vi "Main.vi"(11 "Module Admin":refnum<class "Delacor_lib_QMH_Module Admin.lvclass">) -> ()   [LabVIEW 2020, in "UI.lvlib"]
doc: "This template is based off of the Queued Message Handler design pattern and the Queued Message Handler project template that ships with LabVIEW.\n\nThe main difference is that the queue is private to this module and communication between modules is performed via Broadcast and Request events.\n\nRequest events are wrapped in public API methods and are handled in the Event Handling Loop (EHL) of this VI. Any module can register for Broadcast events sent by this module. The EHL generates messages based on user interface actions.\n\nThe Message Handling Loop (MHL) processes messages generated by the EHL, or by other messages. The messages are string values, so new messages can be added easily to the Message Cases case structure in the MHL. Each message cluster can also provide an optional value for Message Data, which is a variant that can be converted to whatever message-specific data is required.\n_____\nBased on DQMH Dev Tools: Project Template 7.1.2.1547."
uses:
  UI.lvlib
  <vilib>/Delacor/Delacor QMH/Libraries/Module Admin_class/Delacor_lib_QMH_Module Admin.lvclass
  <vilib>/Delacor/Delacor QMH/Libraries/Message Queue_class/Delacor_lib_QMH_Message Queue.lvclass/Delacor_lib_QMH_Message Queue.ctl
  <vilib>/Delacor/Delacor QMH/Libraries/Module Admin_class/Delacor_lib_QMH_Module Admin.lvclass/Delacor_lib_QMH_Module Admin.ctl
  <vilib>/Delacor/Delacor QMH/Libraries/Message Queue_class/Delacor_lib_QMH_Message Queue.lvclass
  Module Data--cluster.ctl
  <vilib>/Utility/miscctls.llb/LVPointTypeDef.ctl
  <vilib>/Delacor/Delacor QMH/Libraries/Message Queue_class/Delacor_lib_QMH_Enqueue Message (Single).vi
  Stop Argument--cluster.ctl
  Get Analog Data Argument--cluster.ctl
panel:
  out "Value":dbl[](array[numeric])
  in  "Start/Stop":bool
  in  "Close":bool
  in  "DAQmx Analog Channels":tag[](array[tag])
  out "error out":errorcluster
  out "Status":string
  in  "Simulate MHL Error":bool
  in  "Simulate EHL Error":bool
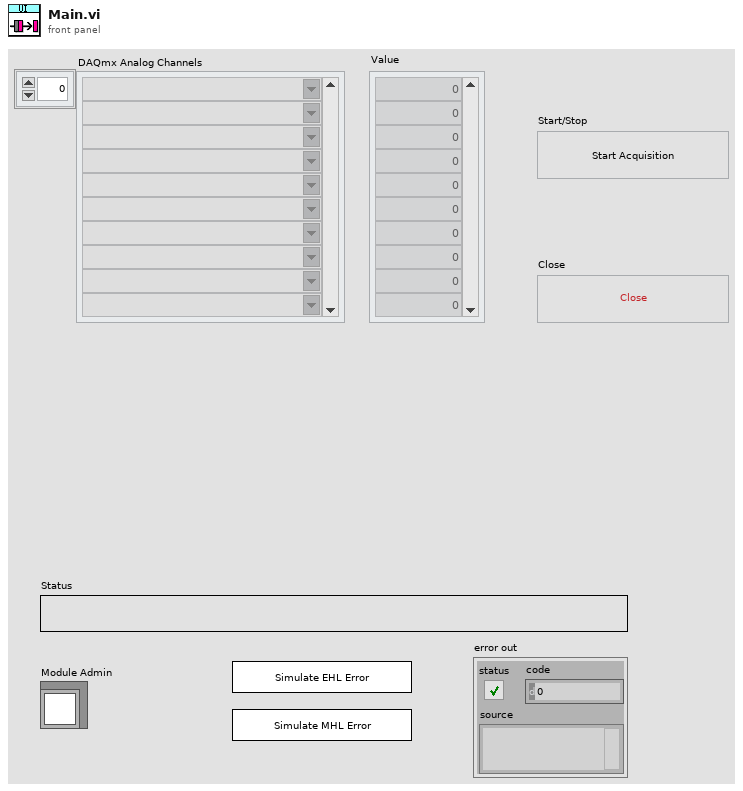
[diagram p1: front panel]
types:
  T1 = typedef "UI.lvlib/Request Events--cluster.ctl" = cluster{"Stop Module":refnum<user-event>, "Show Panel":refnum<user-event>, "Hide Panel":refnum<user-event>, "Get Module Execution Status":refnum<user-event>, "Show Diagram":refnum<user-event>, "Get Analog Data":refnum<user-event>}
  T2 = typedef "UI.lvlib/Module Data--cluster.ctl" = cluster{"Status":string, "Value":dbl[]}
  T3 = enum32{"invalid lock state", "Not Locked", "Locked (No Password)", "Password-protected"}
  T4 = typedef "UI.lvlib/Stop Argument--cluster.ctl" = cluster{"Origin":string, "Exit via Stop Module Req?":bool, "Wait for Module to stop?":bool}
  T5 = typedef "UI.lvlib/Get Analog Data Argument--cluster.ctl" = cluster{"Index":i32, "Value":dbl}
  T6 = enum8{"Enabled", "Disabled", "Disabled and Grayed Out"}
  T7 = typedef "LVPointTypeDef.ctl" = cluster{"Horizontal":i16, "Vertical":i16}
  T8 = enum32{"Invalid", "Standard", "Closed", "Hidden", "Minimized", "Maximized"}
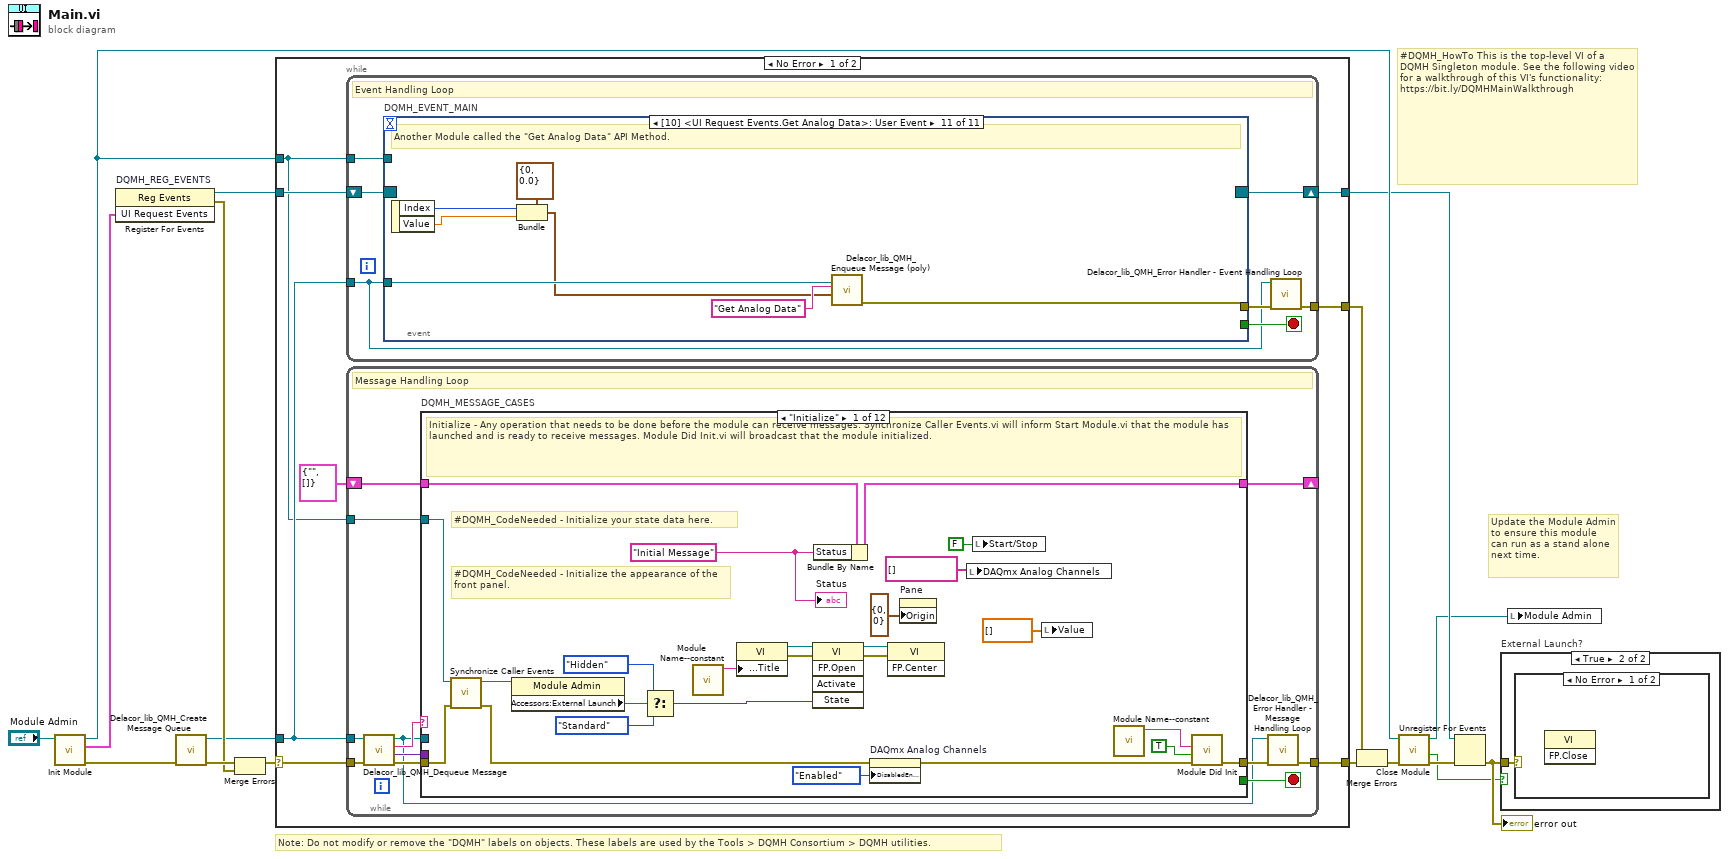
[diagram p0: block diagram]
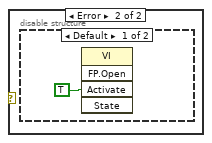
[diagram p3: hidden frame]
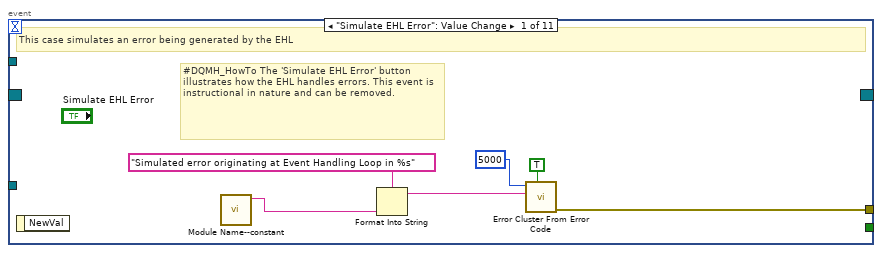
[diagram p5: hidden frame]
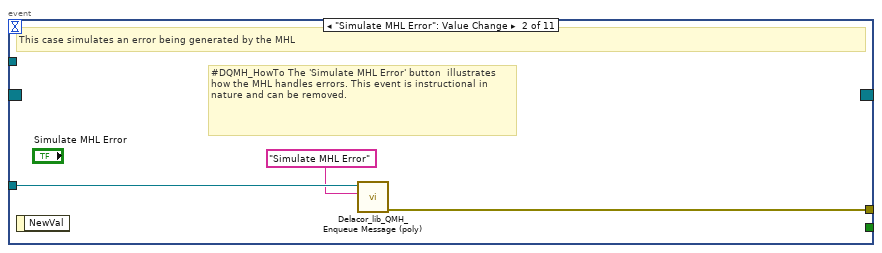
[diagram p6: hidden frame]
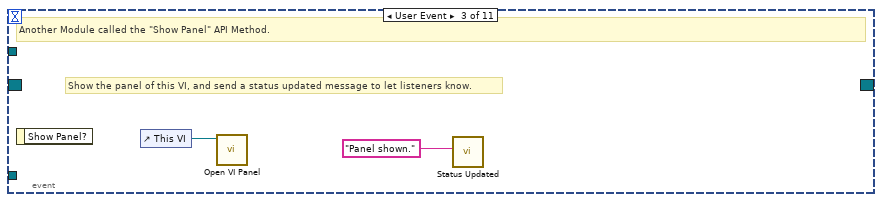
[diagram p7: hidden frame]
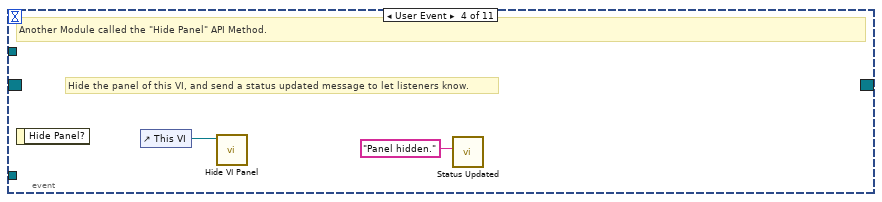
[diagram p8: hidden frame]
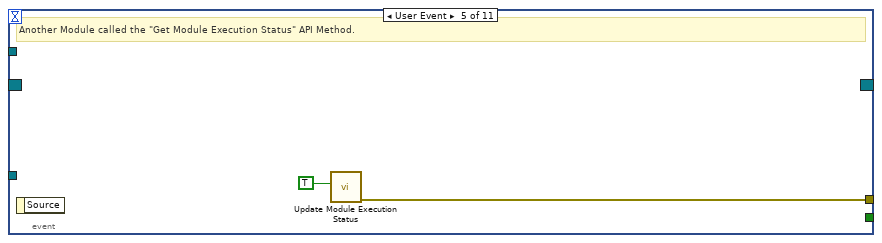
[diagram p9: hidden frame]
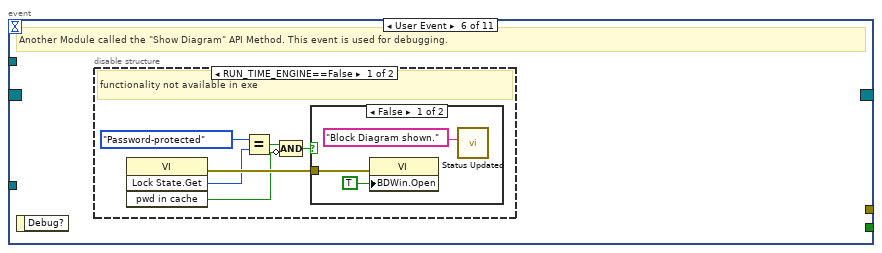
[diagram p10: hidden frame]
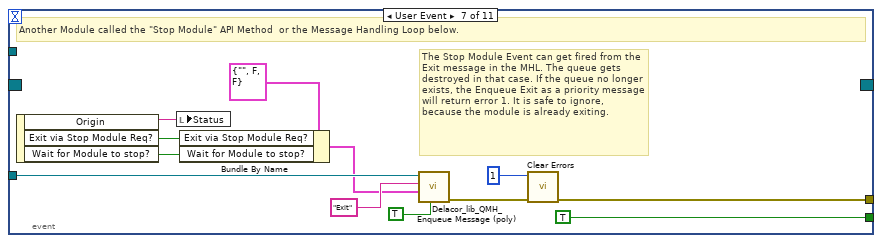
[diagram p13: hidden frame]
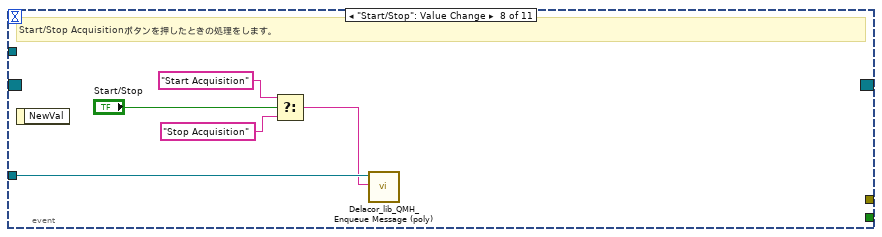
[diagram p14: hidden frame]
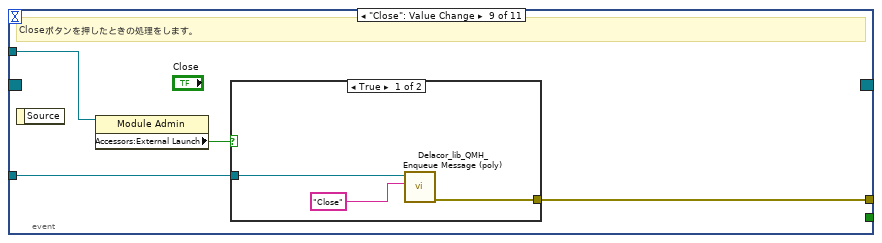
[diagram p15: hidden frame]
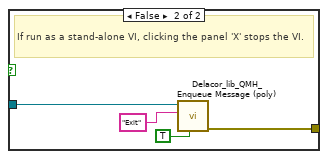
[diagram p16: hidden frame]
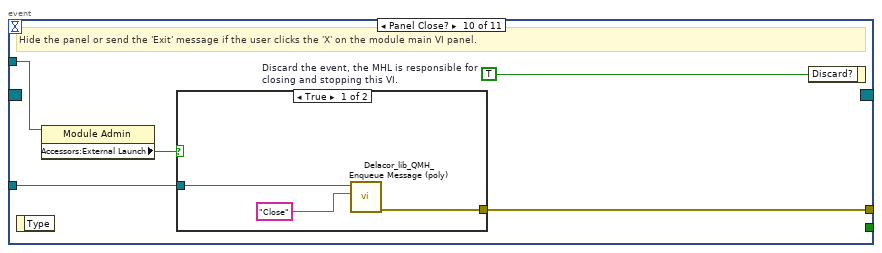
[diagram p17: hidden frame]
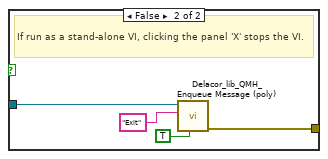
[diagram p18: hidden frame]
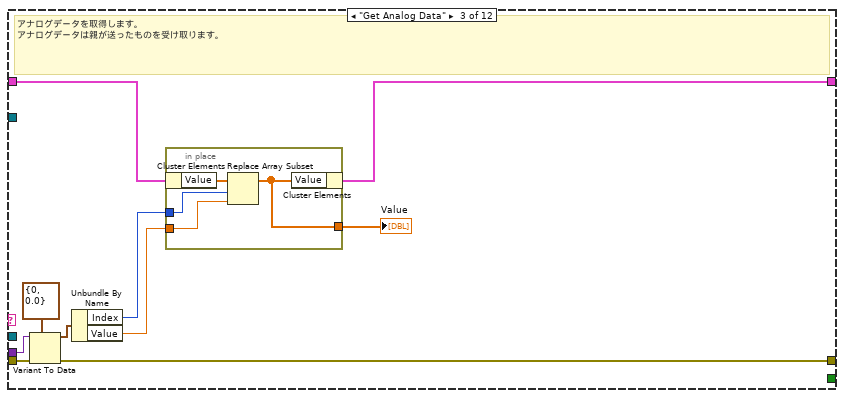
[diagram p20: hidden frame]
diagram:
  # "#DQMH_HowTo This is the top-level VI of a DQMH Singleton module. See the following video for a walkthrough of this VI's functionality: https://bit.ly/DQMHMainWalkthrough"
  # "Note: Do not modify or remove the \"DQMH\" labels on objects. These labels are used by the Tools > DQMH Consortium > DQMH utilities."
  # "Update the Module Admin to ensure this module can run as a stand alone next time."
  n1 = call "Init Module.vi"("Singleton Module Admin in"="Module Admin") -> ("error out"=w16:errorcluster, "UI Request Events"=w5:T1, "Singleton Module Admin out"=w8:refnum<class "Delacor_lib_QMH_Module Admin.lvclass">)  [unwired: 8 in]
  n2 = register-events "DQMH_REG_EVENTS"(w5) -> (reference out=w6:refnum<event-registration>, error out=w9:errorcluster)  [unwired: 2 in]
  n3 = call <vilib>:"Delacor_lib_QMH_Create Message Queue.vi"("error in"=w16) -> ("error out"=w11:errorcluster, "Message Queue"=w4:refnum<class "Delacor_lib_QMH_Message Queue.lvclass">)  [unwired: 9 in]
  n4 = Merge Errors(w11, w9) -> (w10:errorcluster)
  n5 = case shown="No Error" w10 {
    selector: w10 -> [w23 w243]
    tunnel: [w25 w242] -> w17
    tunnel: [w22 w241] -> w7
    tunnel: w6 -> [w20 w241]
    tunnel: w4 -> [w19 w236]
    tunnel: [w24 _] -> w14
    tunnel: w8 -> [w18 w237]
    frame No Error {
      n6 = while {
        tunnel: w19 -> [w26]
        shift-right: [w29] -> w22
        shift-left: w20 -> [w30]
        tunnel: [w31] -> w24
        tunnel: w18 -> [w27]
        stop <- w28 stop-if-true
        # "Event Handling Loop"
        n7 = event "DQMH_EVENT_MAIN" shown="[10] <UI Request Events.Get Analog Data>: User Event" {
          selector: w30 -> [_ _ _ _ _ _ _ _ _ _ _]
          dyn-events: [_ _ _ _ _ _ _ _ _ _ _] -> w29
          timeout: _ -> [_ _ _ _ _ _ _ _ _ _ _]
          tunnel: [_ _ _ _ _ _ TRUE ("Discard?") _ _ _ _] -> w28
          tunnel: w26 -> [_ w40 _ _ _ _ w64 w73 w76 w87 w103]
          tunnel: [w38 w41 _ _ w47 _ w67 _ w74 w89 w97] -> w32
          tunnel: w27 -> [_ _ _ _ _ _ _ _ w75 w86 _]
          event "Simulate EHL Error": Value Change {
            # "#DQMH_HowTo The 'Simulate EHL Error' button  illustrates how the EHL handles errors. This event is instructional in nature and can be removed."
            # "This case simulates an error being generated by the EHL"
            n8 = event-data() -> ()  [unwired: 1 in, 1 out]
            n9 = call "Module Name--constant.vi"() -> ("Module Name"=w35:string)  [unwired: 11 in]
            n10 = Format Into String(format string="Simulated error originating at Event Handling Loop in %s", w35) -> (resulting string=w36:string)  [unwired: 2 in, 1 out]
            n11 = call <vilib>:"Error Cluster From Error Code.vi"("show call chain? (False)"=TRUE, "error message (\"\")"=w36, "error code (0)"=5000) -> ("error out"=w38:errorcluster)  [unwired: 6 in]
          }
          event "Simulate MHL Error": Value Change {
            # "#DQMH_HowTo The 'Simulate MHL Error' button  illustrates how the MHL handles errors. This event is instructional in nature and can be removed."
            # "This case simulates an error being generated by the MHL"
            n12 = event-data() -> ()  [unwired: 1 in, 1 out]
            n13 = call-poly <vilib>:"Delacor_lib_QMH_Enqueue Message (poly).vi"("Message"="Simulate MHL Error", "Message Queue in"=w40) -> ("error out"=w41:errorcluster)  [unwired: 8 in, 1 out]
          }
          event User Event {
            # "Show the panel of this VI, and send a status updated message to let listeners know."
            # "Another Module called the \"Show Panel\" API Method."
            n14 = event-data() -> ()  [unwired: 1 in, 1 out]
            n15 = control-ref of="This VI"() -> (w43:refnum<vi>)
            n16 = call "Open VI Panel.vi"("VI"=w43) -> ()  [unwired: 10 in, 1 out]
            n17 = call "Status Updated.vi"("Status"="Panel shown." ("format string")) -> ()  [unwired: 10 in, 1 out]
          }
          event User Event {
            # "Hide the panel of this VI, and send a status updated message to let listeners know."
            # "Another Module called the \"Hide Panel\" API Method."
            n18 = event-data() -> ()  [unwired: 1 in, 1 out]
            n19 = control-ref of="This VI"() -> (w45:refnum<vi>)
            n20 = call "Hide VI Panel.vi"("VI"=w45) -> ()  [unwired: 10 in, 1 out]
            n21 = call "Status Updated.vi"("Status"="Panel hidden." ("format string")) -> ()  [unwired: 10 in, 1 out]
          }
          event User Event {
            # "Another Module called the \"Get Module Execution Status\" API Method."
            n22 = event-data() -> ()  [unwired: 1 in, 1 out]
            n23 = call "Update Module Execution Status.vi"("Running?"=TRUE) -> ("error out"=w47:errorcluster)  [unwired: 10 in]
          }
          event User Event {
            # "Another Module called the \"Show Diagram\" API Method. This event is used for debugging."
            n24 = event-data() -> ()  [unwired: 1 in, 1 out]
            n25 = disable-structure shown="RUN_TIME_ENGINE==False" {
              frame condition #0 (active) {
                # "functionality not available in exe"
                n26 = invoke on="Invoke Node" class="VI" method="Lock State.Get"() -> (error out=w53:errorcluster, "Get Lock State"=w52:T3, "pwd in cache"=w49:bool)  [unwired: 4 in, 1 out]
                n27 = Equal?(x=T3."Password-protected", y=w52) -> (x = y?=w50:bool)
                n28 = Compound Arithmetic op=AND(w50, invert w49) -> (w48:bool)
                n29 = case shown="False" w48 {
                  tunnel: w53 -> [w56 _]
                  frame False {
                    n30 = property on="Property Node" class="VI"(error in=w56, "BDWin.Open"=TRUE ("Block Diagram Window:Open")) -> ()  [unwired: 1 in, 2 out]
                    n31 = call "Status Updated.vi"("Status"="Block Diagram shown." ("format string")) -> ()  [unwired: 10 in, 1 out]
                  }
                  frame True {
                    # "Password-protected VI, and the password is not in the cache. Do not show the diagram."
                  }
                }
              }
              frame condition #1 {
              }
            }
          }
          event User Event {
            # "The Stop Module Event can get fired from the Exit message in the MHL. The queue gets destroyed in that case. If the queue no longer exists, the Enqueue Exit as a priority message will return error 1. It is safe to ignore, because the module is already exiting."
            # "Another Module called the \"Stop Module\" API Method  or the Message Handling Loop below."
            n32 = event-data() -> ("Origin"=w63:string, "Exit via Stop Module Req?"=w59:bool, "Wait for Module to stop?"=w58:bool)  [unwired: 1 in]
            n33 = local write "Status"(w63) -> ()
            n34 = Bundle By Name(cluster=T4 {"Origin"="", "Exit via Stop Module Req?"=FALSE, "Wait for Module to stop?"=FALSE} ("Stop Argument"), "Exit via Stop Module Req?"=w59, "Wait for Module to stop?"=w58) -> (w57:T4)
            n35 = call-poly <vilib>:"Delacor_lib_QMH_Enqueue Message (poly).vi"("Priority Message? (F)"=TRUE, "Message Data"=w57, "Message"="Exit", "Message Queue in"=w64) -> ("error out"=w68:errorcluster)  [unwired: 6 in, 1 out]
            n36 = call <vilib>:"Clear Errors.vi"("error in (no error)"=w68, "specific error code to clear (0: all)"=1) -> ("error out"=w67:errorcluster)  [unwired: 4 in, 1 out]
          }
          event "Start/Stop": Value Change {
            # "Start/Stop Acquisitionボタンを押したときの処理をします。"
            n37 = event-data() -> ()  [unwired: 1 in, 1 out]
            n38 = Select(t="Start Acquisition" ("Message"), s="Start/Stop", f="Stop Acquisition" ("Message")) -> (s? t:f=w69:string)
            n39 = call-poly <vilib>:"Delacor_lib_QMH_Enqueue Message (poly).vi"("Message"=w69, "Message Queue in"=w73) -> ()  [unwired: 8 in, 2 out]
          }
          event "Close": Value Change {
            # "Closeボタンを押したときの処理をします。"
            n40 = event-data() -> ()  [unwired: 1 in, 1 out]
            n41 = property on="Property Node" class="Module Admin"(reference=w75) -> ("Accessors:External Launch"=w77:bool)  [unwired: 1 in, 2 out]
            n42 = case shown="True" w77 {
              tunnel: w76 -> [w79 w83]
              tunnel: [w78 w84] -> w74
              frame True {
                n43 = call-poly <vilib>:"Delacor_lib_QMH_Enqueue Message (poly).vi"("Message"="Close", "Message Queue in"=w79) -> ("error out"=w78:errorcluster)  [unwired: 8 in, 1 out]
              }
              frame False {
                # "If run as a stand-alone VI, clicking the panel 'X' stops the VI."
                n44 = call-poly <vilib>:"Delacor_lib_QMH_Enqueue Message (poly).vi"("Priority Message? (F)"=TRUE, "Message"="Exit", "Message Queue in"=w83) -> ("error out"=w84:errorcluster)  [unwired: 7 in, 1 out]
              }
            }
          }
          event Panel Close? {
            w88 = TRUE  # Discard the event, the MHL is responsible for closing and stopping this VI.
            # "Hide the panel or send the 'Exit' message if the user clicks the 'X' on the module main VI panel."
            n45 = event-data() -> ()  [unwired: 1 in, 1 out]
            n46 = property on="Property Node" class="Module Admin"(reference=w86) -> ("Accessors:External Launch"=w85:bool)  [unwired: 1 in, 2 out]
            n47 = case shown="True" w85 {
              tunnel: w87 -> [w91 w95]
              tunnel: [w90 w96] -> w89
              frame True {
                n48 = call-poly <vilib>:"Delacor_lib_QMH_Enqueue Message (poly).vi"("Message"="Close", "Message Queue in"=w91) -> ("error out"=w90:errorcluster)  [unwired: 8 in, 1 out]
              }
              frame False {
                # "If run as a stand-alone VI, clicking the panel 'X' stops the VI."
                n49 = call-poly <vilib>:"Delacor_lib_QMH_Enqueue Message (poly).vi"("Priority Message? (F)"=TRUE, "Message"="Exit", "Message Queue in"=w95) -> ("error out"=w96:errorcluster)  [unwired: 7 in, 1 out]
              }
            }
            n50 = event-data ("Event Filter Node")("Discard?"=w88) -> ()  [unwired: 1 in, 1 out]
          }
          event User Event {
            # "Another Module called the \"Get Analog Data\" API Method."
            n51 = event-data() -> ("Index"=w99:i32, "Value"=w98:dbl)  [unwired: 1 in]
            n52 = Bundle(cluster=T5 {"Index"=0, "Value"=0.0} ("Get Analog Data Argument"), "Index"=w99, "Value"=w98) -> (w100:T5)
            n53 = call-poly <vilib>:"Delacor_lib_QMH_Enqueue Message (poly).vi"("Message Data"=w100, "Message"="Get Analog Data", "Message Queue in"=w103) -> ("error out"=w97:errorcluster)  [unwired: 7 in, 1 out]
          }
        }
        n54 = call-dynamic "Delacor_lib_QMH_Error Handler - Event Handling Loop.vi"("error in"=w32, "Message Queue in"=w26) -> ("dup error in"=w31:errorcluster)  [unwired: 8 in, 1 out]
      }
      n55 = while {
        tunnel: w19 -> [w104]
        shift-right: [w112] -> _
        shift-left: T2 {"Status"="", "Value"=[]} ("Data Cluster") -> [w113]
        tunnel: w23 -> [w115]
        tunnel: [w107] -> w25
        tunnel: w18 -> [w108]
        stop <- w111 stop-if-true
        # "Message Handling Loop"
        n56 = call-dynamic "Delacor_lib_QMH_Dequeue Message.vi"("error in"=w115, "Message Queue in"=w104) -> ("error out"=w114:errorcluster, "Message Data"=w109:variant, "Message"=w110:string, "Message Queue out"=w105:refnum<class "Delacor_lib_QMH_Message Queue.lvclass">)  [unwired: 6 in]
        n57 = case "DQMH_MESSAGE_CASES" shown="\"Initialize\"" w110 {
          selector: w110 -> [_ _ _ _ _ _ _ _ _ _ _ w231]
          tunnel: w105 -> [_ _ _ _ _ _ _ _ _ w197 w219 _]
          tunnel: w114 -> [w138 w142 w152 w159 w169 w175 w178 w184 w193 w204 w225 w234]
          tunnel: [w137 w142 w151 w158 w170 w177 w182 w184 w192 w200 w220 w235] -> w106
          tunnel: w113 -> [w128 w141 w147 w157 w165 w176 w181 w183 w190 w199 w218 w232]
          tunnel: [w127 w141 w146 w157 w164 w176 w181 w183 w190 w199 w218 w232] -> w112
          tunnel: [_ _ _ _ _ _ _ _ _ _ w217 _] -> w111
          tunnel: w109 -> [_ _ w150 _ _ _ _ _ _ w198 w216 _]
          tunnel: w108 -> [w129 _ _ _ _ _ _ _ _ w196 w211 _]
          frame "Initialize" {
            w123 = "Initial Message" ("Initial Message")
            # "#DQMH_CodeNeeded - Initialize the appearance of the front panel."
            # "#DQMH_CodeNeeded - Initialize your state data here."
            # "Initialize - Any operation that needs to be done before the module can receive messages. Synchronize Caller Events.vi will inform Start Module.vi that the module has launched and is ready to receive messages. Module Did Init.vi will broadcast that the module initialized."
            n58 = call "Synchronize Caller Events.vi"("error in"=w138, "Singleton Module Admin in"=w129) -> ("error out"=w120:errorcluster, "Singleton Module Admin out"=w124:refnum<class "Delacor_lib_QMH_Module Admin.lvclass">)  [unwired: 8 in]
            n59 = property on="Property Node" class="Module Admin"(reference=w124) -> ("Accessors:External Launch"=w133:bool)  [unwired: 1 in, 2 out]
            n60 = Select(t=T8."Hidden" ("State"), s=w133, f=T8."Standard" ("State")) -> (s? t:f=w130:T8)
            n61 = call "Module Name--constant.vi"() -> ("Module Name"=w136:string)  [unwired: 11 in]
            n62 = property on="Property Node" class="VI"("Front Panel.Title"=w136) -> (reference out=w135:refnum<vi>, error out=w140:errorcluster)  [unwired: 2 in]
            n63 = invoke on="Invoke Node" class="VI" method="FP.Open"(reference=w135, error in=w140, "State"=w130) -> (reference out=w134:refnum<vi>, error out=w139:errorcluster)  [unwired: 2 in, 3 out]
            n64 = Bundle By Name(cluster=w128, "Status"=w123) -> (w127:T2)
            n65 = property on="DAQmx Analog Channels" class="Arr (strict)"(error in=w120, "DisabledEnum"=T6."Enabled" ("Disabled")) -> (error out=w119:errorcluster)  [unwired: 1 in, 1 out]
            n66 = invoke on="Invoke Node" class="VI" method="FP.Center"(reference=w134, error in=w139) -> ()  [unwired: 1 in, 3 out]
            n67 = property on="Pane" class="Pane"("Origin"=T7 {"Horizontal"=0, "Vertical"=0}) -> ()  [unwired: 2 in, 2 out]
            n68 = local write "DAQmx Analog Channels"(tag[] [] ("DAQmx Analog Channels")) -> ()
            n69 = local write "Start/Stop"(FALSE ("Start/Stop")) -> ()
            n70 = local write "Value"(dbl[] [] ("Value")) -> ()
            n71 = call "Module Name--constant.vi"() -> ("Module Name"=w125:string)  [unwired: 11 in]
            n72 = call "Module Did Init.vi"("error in"=w119, "Initialized?"=TRUE, "Origin"=w125) -> ("error out"=w137:errorcluster)  [unwired: 8 in]
            "Status" <- w123
          }
          frame "---Module Specific---" {
            # "Separator -- The following cases handle messages specific to this Module."
          }
          frame "Get Analog Data" {
            # "アナログデータを取得します。\nアナログデータは親が送ったものを受け取ります。"
            n73 = Variant To Data(error in=w152, type=T5 {"Index"=0, "Value"=0.0} ("Get Analog Data Argument"), Variant=w150) -> (data=w148:T5, error out=w151:errorcluster)
            n74 = Unbundle By Name(w148) -> ("Index"=w145:i32, "Value"=w144:dbl)
            n75 = in-place {
              in-place-border: w145 -> [w155]
              in-place-border: w144 -> [w154]
              in-place-border: [w153] -> w143
              n76 = in-place-cluster #1(w147) -> ("Value"=w156:dbl[])
              n77 = Replace Array Subset(array=w156, new element=w154, index=w155) -> (w153:dbl[])
              n78 = in-place-cluster #1("Value"=w153) -> (w146:T2)
            }
            "Value" <- w143
          }
          frame "---Copy This Frame---" {
            # "Duplicate this frame when creating new messages.  Change this comment in the duplicated frame to describe this message."
            n79 = Merge Errors(w159) -> (w158:errorcluster)
          }
          frame "Start Acquisition" {
            # "集録開始の処理を親に送ります。\nDAQ物理チャンネルを送った後にこの制御器の操作を無効にします。"
            n80 = Array Size(array="DAQmx Analog Channels") -> (size(s)=w162:i32)
            n81 = call "Start Acquisition.vi"("error in"=w169, "DAQmx Analog Channels"="DAQmx Analog Channels") -> ("error out"=w168:errorcluster)  [unwired: 9 in]
            n82 = Initialize Array(0.0 ("Numeric"), w162) -> (w160:dbl[])
            n83 = Bundle By Name(cluster=w165, "Value"=w160) -> (w164:T2)
            n84 = property on="DAQmx Analog Channels" class="Arr (strict)"(error in=w168, "DisabledEnum"=T6."Disabled" ("Disabled")) -> (error out=w167:errorcluster)  [unwired: 1 in, 1 out]
            n85 = Merge Errors(w167) -> (w170:errorcluster)
          }
          frame "Stop Acquisition" {
            # "集録停止の処理を親に送ります。\nDAQ物理チャンネルを送った後にこの制御器の操作を有効にします。"
            n86 = call "Stop Acquisition.vi"("error in"=w175, "Boolean"=FALSE) -> ("error out"=w172:errorcluster)  [unwired: 9 in]
            n87 = property on="DAQmx Analog Channels" class="Arr (strict)"(error in=w172, "DisabledEnum"=T6."Enabled" ("Disabled")) -> (error out=w173:errorcluster)  [unwired: 1 in, 1 out]
            n88 = Merge Errors(w173) -> (w177:errorcluster)
          }
          frame "Close" {
            # "アプリケーション終了の指示を親に送ります。\nこの時点ではこのモジュールは終了しません。\n親からExitの指示をもらったら終了します。"
            n89 = call "Close.vi"("error in"=w178, "Dummy"=TRUE ("Boolean")) -> ("error out"=w179:errorcluster)  [unwired: 9 in]
            n90 = Merge Errors(w179) -> (w182:errorcluster)
          }
          frame "---Exit and Error Handling---" {
            # "Separator - The following cases handle errors and exit messages."
          }
          frame "Simulate MHL Error" {
            # "#DQMH_HowTo The 'Simulate MHL Error' button  illustrates how the MHL handles errors. This event is instructional in nature and can be removed."
            # "Simulate an error occurring at the MHL"
            n91 = call "Module Name--constant.vi"() -> ("Module Name"=w186:string)  [unwired: 11 in]
            n92 = Format Into String(format string="Simulated error originating at Message Handling Loop in %s", w186) -> (resulting string=w187:string)  [unwired: 2 in, 1 out]
            n93 = call <vilib>:"Error Cluster From Error Code.vi"("show call chain? (False)"=TRUE, "error message (\"\")"=w187, "error code (0)"=5001) -> ("error out"=w191:errorcluster)  [unwired: 6 in]
            n94 = Merge Errors(w193, w191) -> (w192:errorcluster)
          }
          frame "Error" {
            # "#DQMH_CodeRecommended - If the module is running in standalone mode (External Launch = FALSE), this code will pop up an error dialog and call the 'Exit' message if an error occurs. Add more fine-grained error management here."
            # "Error - Check the error message data and respond accordingly. This message is sent by the \"Error Handler\" VIs at the end of each loop in this application."
            n95 = property on="Property Node" class="Module Admin"(reference=w196) -> ("Accessors:External Launch"=w195:bool)  [unwired: 1 in, 2 out]
            n96 = Variant To Data(error in=w204, type=errorcluster {"status"=FALSE, "code"=0, "source"=""} ("error constant"), Variant=w198) -> (data=w194:errorcluster, error out=w202:errorcluster)
            n97 = local write "error out"(w194) -> ()
            n98 = call "Error Reported.vi"("Error"=w194) -> ()  [unwired: 10 in, 1 out]
            n99 = case shown="False" w195 {
              tunnel: [w209 _] -> w201
              tunnel: w197 -> [w207 _]
              tunnel: w194 -> [w208 _]
              frame False {
                n100 = disable-structure shown="DQMH_Disable_SEH==TRUE" {
                  disable-tunnel: w208 -> [w210 _]
                  frame condition #0 {
                    # "If the module is running standalone, then pop up an error dialog and call the \"Exit\" message."
                    n101 = call <vilib>:"Simple Error Handler.vi"("error in (no error)"=w210) -> ()  [unwired: 4 in, 5 out]
                  }
                  frame condition #1 (active) {
                    # "To prevent the Simple Error Handler VI from being loaded (e.g. when deploying to a Real-Time target), add the Conditional Disable Symbol \"DQMH_Disable_SEH\" to your project and set it to TRUE."
                  }
                }
                n102 = call-poly <vilib>:"Delacor_lib_QMH_Enqueue Message (poly).vi"("Priority Message? (F)"=TRUE, "Message"="Exit", "Message Queue in"=w207) -> ("error out"=w209:errorcluster)  [unwired: 7 in, 1 out]
              }
              frame True {
                # "If the module was launched externally, calling the Error Reported broadcast VI is the only action performed by the \"Error\" message. The module's caller can then process the error appropriately."
              }
            }
            n103 = Merge Errors(w202, w201) -> (w200:errorcluster)
          }
          frame "Exit" {
            w215 = 91  # 91: not all Exit messages will have an argument
            w217 = TRUE  # Stop the VI
            # "Release the message queue reference"
            # "#DQMH_CodeNeeded - Add any required cleanup code here."
            # "Exit - Exit the application."
            n104 = Variant To Data(error in=w225, type=T4 {"Origin"="", "Exit via Stop Module Req?"=FALSE, "Wait for Module to stop?"=FALSE} ("Stop Argument"), Variant=w216) -> (data=w213:T4, error out=w222:errorcluster)
            n105 = call <vilib>:"Clear Errors.vi"("error in (no error)"=w222, "specific error code to clear (0: all)"=w215) -> ("error out"=w224:errorcluster)  [unwired: 4 in, 1 out]
            n106 = control-ref of="This VI"() -> (w212:refnum<vi>)
            n107 = call-dynamic "Delacor_lib_QMH_Release Message Queue.vi"("error in"=w224, "Message Queue"=w219) -> ("error out"=w223:errorcluster)  [unwired: 9 in]
            n108 = call "Handle Exit.vi"("Stop Argument"=w213, "Admin in"=w211, "VI reference"=w212) -> ("error out"=w221:errorcluster)  [unwired: 7 in, 1 out]
            n109 = Merge Errors(w223, w221) -> (w220:errorcluster)
            n110 = call "Error Reported.vi"("Error"=w220) -> ()  [unwired: 10 in, 1 out]
          }
          frame Default {
            # "'Default' case only runs if there is a message that isn't defined in any of the other cases.  Output a programming error."
            n111 = call "Module Name--constant.vi"() -> ("Module Name"=w230:string)  [unwired: 11 in]
            n112 = Format Into String(format string="The invalid message string \"%s\" was received in the Message Handling Loop for module \"%s\".", w231, w230) -> (resulting string=w226:string)  [unwired: 2 in, 1 out]
            n113 = call <vilib>:"Error Cluster From Error Code.vi"("show call chain? (False)"=TRUE, "error message (\"\")"=w226, "error code (0)"=1) -> ("error out"=w233:errorcluster)  [unwired: 6 in]
            n114 = Merge Errors(w234, w233) -> (w235:errorcluster)
          }
        }
        n115 = call-dynamic "Delacor_lib_QMH_Error Handler - Message Handling Loop.vi"("error in"=w106, "Message Queue in"=w105) -> ("dup error in"=w107:errorcluster)  [unwired: 8 in, 1 out]
      }
    }
    frame Error {
      # "Synchronize Caller Events.vi will inform Start Module.vi that the module has launched and will let the code calling Start Module.vi register for broadcasts and would permit the caller receive the broadcast that an error occurred at launch time."
      n116 = call-dynamic "Delacor_lib_QMH_Release Message Queue.vi"("error in"=w243, "Message Queue"=w236) -> ("error out"=w242:errorcluster)  [unwired: 9 in]
      n117 = call "Synchronize Caller Events.vi"("Singleton Module Admin in"=w237) -> ("error out"=w244:errorcluster)  [unwired: 9 in, 1 out]
      n118 = call "Module Name--constant.vi"() -> ("Module Name"=w240:string)  [unwired: 11 in]
      n119 = Format Into String(format string="An error occurred during initialization. %s is no longer running.", w240) -> (resulting string=w238:string)  [unwired: 2 in, 1 out]
      n120 = Merge Errors(w242, w244) -> (w245:errorcluster)
      n121 = call "Error Reported.vi"("Additional Information"=w238, "Error"=w245) -> ()  [unwired: 9 in, 1 out]
    }
  }
  n122 = Merge Errors(w14, w17) -> (w13:errorcluster)
  n123 = call "Close Module.vi"("error in"=w13, "Module Admin in"=w8) -> ("error out"=w15:errorcluster, "External Launch"=w1:bool, "Module Admin out"=w2:refnum<class "Delacor_lib_QMH_Module Admin.lvclass">)  [unwired: 7 in]
  n124 = Unregister For Events(event registration refnum=w7, error in=w15) -> (error out=w12:errorcluster)
  "error out" <- w12
  n125 = case "External Launch?" shown="True" w1 {
    tunnel: w12 -> [_ w246]
    frame False {
    }
    frame True {
      n126 = case shown="No Error" w246 {
        frame No Error {
          n127 = invoke on="Invoke Node" class="VI" method="FP.Close"() -> ()  [unwired: 3 in, 3 out]
        }
        frame Error {
          n128 = disable-structure shown="Default" {
            frame condition #0 (active) {
              n129 = invoke class="VI" method="FP.Open"("Activate"=TRUE ("Activate?")) -> ()  [unwired: 4 in, 5 out]
            }
            frame condition #1 {
              # "Don't show panel on error if running inside a built EXE."
            }
          }
        }
      }
    }
  }
  n130 = local write "Module Admin"(w2) -> ()
